vi "Max Block Count (Transfer Group).vi"(8 "error in (no error)":errorcluster, 10 "largest block count in (0)":u64, 11 "Transfer Group in":T1={"name"="", "direction"=enum."Tx", "cycle timing"={"priority"=0, "decimation"=1, "offset"=0}, "Transfers"=[], "settings"=[]} {"Transfers"."channels"."dst buffer offset" format="%d bytes"; "Transfers"."channels"."src buffer offset" format="%d bytes"}) -> (0 "error out":errorcluster, 2 "largest block count out":u64, 3 "Transfer out":T1={"name"="", "direction"=enum."Tx", "cycle timing"={"priority"=0, "decimation"=1, "offset"=0}, "Transfers"=[], "settings"=[]} {"Transfers"."channels"."dst buffer offset" format="%d bytes"; "Transfers"."channels"."src buffer offset" format="%d bytes"})   [LabVIEW 2017, in "DSF Core.lvlib"]
uses:
  DSF Core.lvlib
  Controls/DSF Engine Transfer Group Configuration.ctl
  Controls/DSF Direction.ctl
  Controls/DSF Timing Info.ctl
  Controls/DSF Engine Transfer Configuration.ctl
  Controls/DSF Byte Order.ctl
  Controls/DSF Engine Channel Configuration.ctl
  Controls/DSF Data Type.ctl
  Controls/DSF Settings Info.ctl
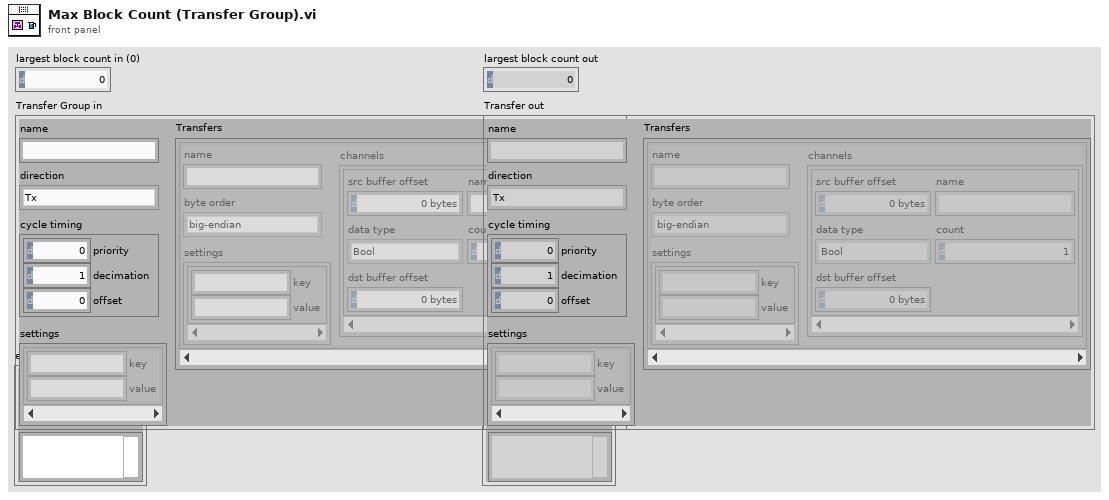
[diagram p1: front panel]
types:
  T1 = typedef "DSF Core.lvlib/DSF Engine Transfer Group Configuration.ctl" = cluster{"name":string, "direction":T2, "cycle timing":T3, "Transfers":T4[], "settings":T8}
  T2 = typedef "DSF Core.lvlib/DSF Direction.ctl" = enum8{"Tx", "Rx"}
  T3 = typedef "DSF Core.lvlib/DSF Timing Info.ctl" = cluster{"priority":u64, "decimation":u64, "offset":u64}
  T4 = typedef "DSF Core.lvlib/DSF Engine Transfer Configuration.ctl" = cluster{"name":string, "byte order":T5, "channels":T6[], "settings":T8}
  T5 = typedef "DSF Core.lvlib/DSF Byte Order.ctl" = enum8{"big-endian", "little-endian"}
  T6 = typedef "DSF Core.lvlib/DSF Engine Channel Configuration.ctl" = cluster{"src buffer offset":u64, "name":string, "data type":T7, "count":u64, "dst buffer offset":u64}
  T7 = typedef "DSF Core.lvlib/DSF Data Type.ctl" = enum8{"Bool", "SGL", "DBL", "I8", "I16", "I32", "I64", "U8", "U16", "U32", "U64"}
  T8 = typedef "DSF Core.lvlib/DSF Settings Info.ctl" = cluster{"key":string, "value":string}[]
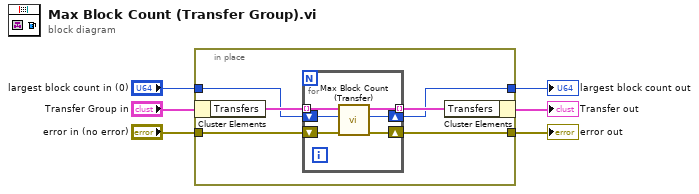
[diagram p0: block diagram]
diagram:
  n1 = in-place {
    in-place-border: "error in (no error)" -> [w10]
    in-place-border: [w9] -> w4
    in-place-border: "largest block count in (0)" -> [w8]
    in-place-border: [w7] -> w1
    n2 = in-place-cluster #1("Transfer Group in") -> ("Transfers"=w12:T4[])
    n3 = for {
      tunnel: w12 -> [w18] mode=indexing
      tunnel: [w17] -> w11 mode=indexing
      shift-right: [w15] -> w9
      shift-left: w10 -> [w16]
      shift-right: [w13] -> w7
      shift-left: w8 -> [w14]
      n4 = call "Max Block Count (Transfer).vi"("error in (no error)"=w16, "largest block count in (0)"=w14, "Transfer in"=w18) -> ("error out"=w15:errorcluster, "largest block count out"=w13:u64, "Transfer out"=w17:T4)  [unwired: 6 in]
    }
    n5 = in-place-cluster #1("Transfers"=w11) -> (→"Transfer out":T1)
  }
  "error out" <- w4
  "largest block count out" <- w1
